vi "Acquiring.vi"(4 "Notify":refnum<notifier>, 6 "GrphChrt Refnum":refnum<vi>, 8 "error in":errorcluster, 9 "Processing Queue":refnum<queue>, 10 "Flow Queue":refnum<queue>, 11 "Acquire Queue":refnum<queue>) -> (0 "error out":errorcluster)   [LabVIEW 2016]
uses:
  Queue Message Handler/Message Cluster.ctl
  Control/Settings.ctl
  Control/port config.ctl
  <vilib>/LabVIEW Interface for Arduino/Type Defs/Board Type.ctl
  <vilib>/LabVIEW Interface for Arduino/Type Defs/Arduino Resource.ctl
  Queue Message Handler/Message Queue.lvlib
  <vilib>/LabVIEW Interface for Arduino/LabVIEW Interface for Arduino.lvlib
panel:
  out "delta t":dbl
  out "Waveform Chart":dbl[](graph)
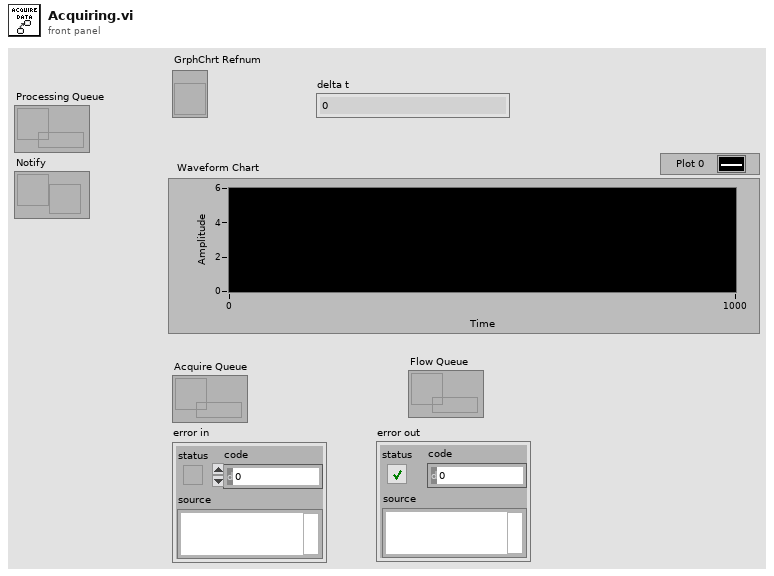
[diagram p1: front panel]
types:
  T1 = typedef "Settings.ctl" = cluster{"Port":T2, "Sample Rate (HZ)":u16, "Samples to Read":u16, "Input Pin":u8, "File path saved":path}
  T2 = typedef "port config.ctl" = cluster{"Port Name":refnum<visa-resource-name>, "Board Type":T3, "Baud Rate":u32}
  T3 = typedef "LabVIEW Interface for Arduino.lvlib/Board Type.ctl" = enum16{"Uno", "Dimuelanove w/Atmega 328", "Mega 2560"}
  T4 = typedef "LabVIEW Interface for Arduino.lvlib/Arduino Resource.ctl" = cluster{"VISA resource":refnum<visa-resource-name>, "Board Type":T3, "Connection Type":enum8{"USB / Serial"}, "Bytes Per Packet (15)":u8}
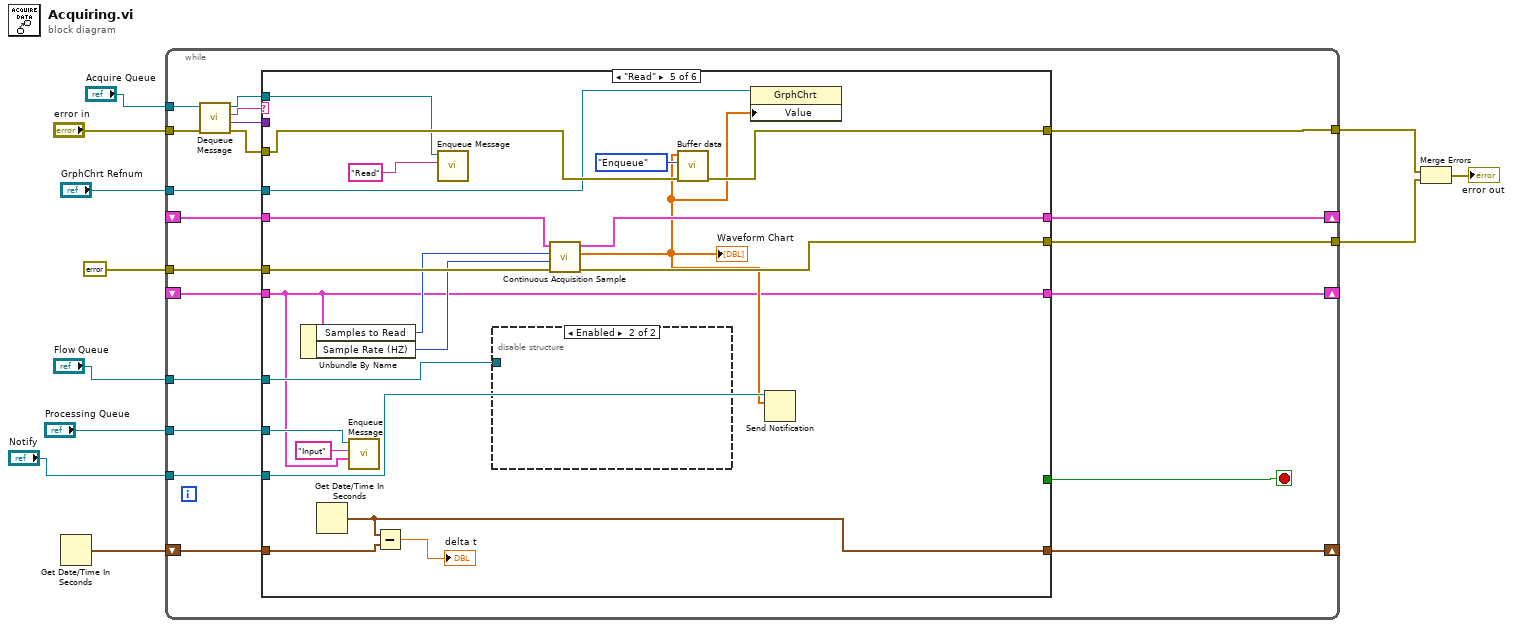
[diagram p0: block diagram]
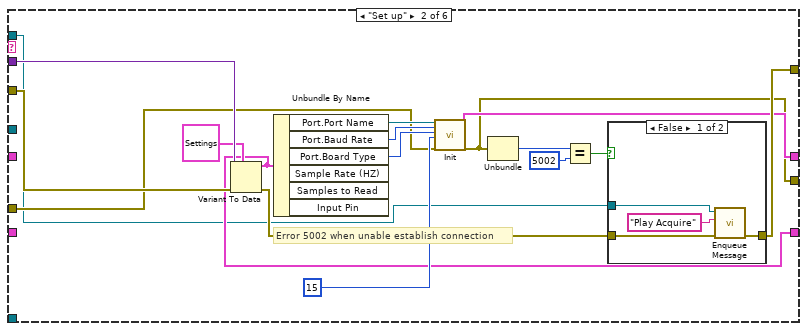
[diagram p3: hidden frame]
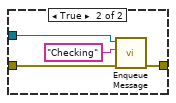
[diagram p4: hidden frame]
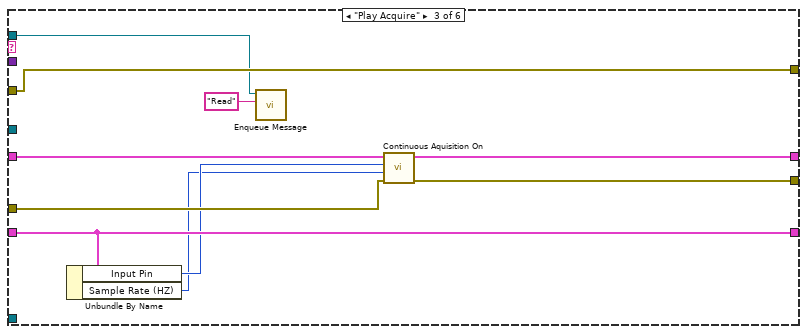
[diagram p5: hidden frame]
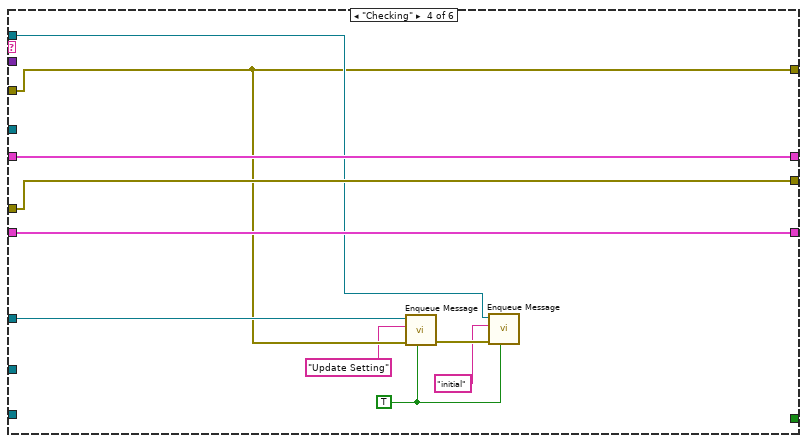
[diagram p6: hidden frame]
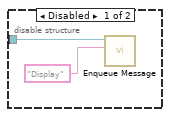
[diagram p7: hidden frame]
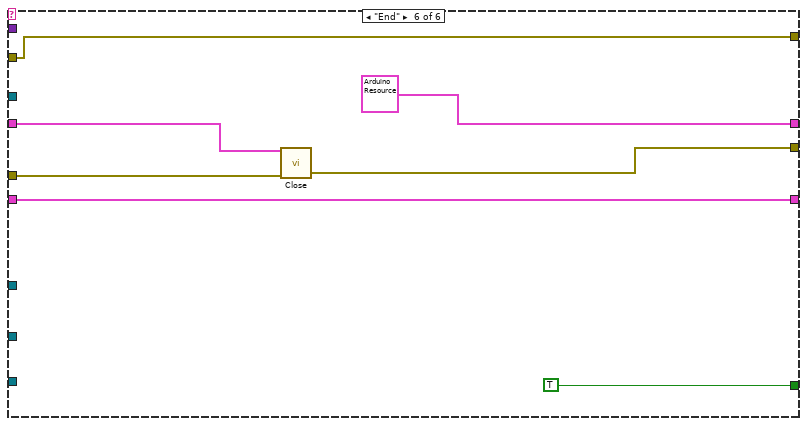
[diagram p8: hidden frame]
diagram:
  n1 = Get Date/Time In Seconds() -> (seconds since 1Jan1904=w1:timestamp)
  n2 = while {
    tunnel: "Acquire Queue" -> [w31]
    tunnel: "error in" -> [w30]
    shift-right: [w25] -> _
    shift-left: _ -> [w24]
    tunnel: [w23] -> w7
    tunnel: errorcluster {"status"=FALSE, "code"=0, "source"=""} ("error in") -> [w22]
    tunnel: [w20] -> w8
    shift-right: [w19] -> _
    shift-left: _ -> [w18]
    tunnel: "Flow Queue" -> [w17]
    tunnel: "GrphChrt Refnum" -> [w16]
    tunnel: "Processing Queue" -> [w15]
    tunnel: "Notify" -> [w14]
    shift-right: [w12] -> _
    shift-left: w1 -> [w13]
    stop <- w28 stop-if-true
    n3 = call "Dequeue Message.vi"("error in (no error)"=w30, "Message Queue"=w31) -> ("error out"=w26:errorcluster, "Message Data"=w27:variant, "Message"=w29:string, "dup Message Queue"=w21:refnum<queue>)  [unwired: 6 in]
    n4 = case shown="\"Read\"" w29 {
      tunnel: [_ _ _ _ _ TRUE] -> w28
      tunnel: w27 -> [_ w52 _ _ _ _]
      tunnel: w26 -> [w33 w46 w70 w75 w94 w109]
      tunnel: [w35 w37 w66 w78 w98 T4 {"VISA resource"="", "Board Type"=enum."Uno", "Connection Type"=enum."USB / Serial", "Bytes Per Packet (15)"=15} ("Arduino Resource")] -> w25
      tunnel: w24 -> [w35 _ w67 w78 w99 w105]
      tunnel: [w34 w36 w64 w80 w100 w106] -> w23
      tunnel: w22 -> [w34 w45 w65 w80 w101 w107]
      tunnel: w21 -> [_ w39 w69 w77 w91 _]
      tunnel: [w33 w38 w70 w75 w93 w109] -> w20
      tunnel: [w32 w44 w63 w79 w81 w108] -> w19
      tunnel: w18 -> [w32 _ w63 w79 w81 w108]
      tunnel: w17 -> [_ _ _ w76 w90 _]
      tunnel: w16 -> [_ _ _ _ w89 _]
      tunnel: w15 -> [_ _ _ _ w88 _]
      tunnel: w14 -> [_ _ _ _ w86 _]
      tunnel: w13 -> [_ _ _ _ w84 _]
      tunnel: [_ _ _ _ w83 _] -> w12
      frame "initial", Default {
      }
      frame "Set up" {
        # "Error 5002 when unable establish connection"
        n5 = Variant To Data(error in=w46, type=T1 {"Port"={"Port Name"="", "Board Type"=enum."Uno", "Baud Rate"=115200}, "Sample Rate (HZ)"=100, "Samples to Read"=50, "Input Pin"=0, "File path saved"=path ""} ("Settings out"), Variant=w52) -> (data=w44:T1, error out=w40:errorcluster)
        n6 = Unbundle By Name(w44) -> ("Port.Port Name"=w50:refnum<visa-resource-name>, "Port.Baud Rate"=w49:u32, "Port.Board Type"=w48:T3)  [unwired: 3 out]
        n7 = call <vilib>:"Init.vi"("VISA resource"=w50, "Baud Rate (115200)"=w49, "Board Type (Uno)"=w48, "Bytes Per Packet (15)"=u32 15, "error in"=w45) -> ("Arduino Resource"=w37:T4, "error out"=w36:errorcluster)  [unwired: 13 in]
        n8 = Unbundle(w36) -> ("code"=w43:i32)  [unwired: 2 out]
        n9 = Equal?(x=w43, y=5002) -> (x = y?=w41:bool)
        n10 = case shown="False" w41 {
          tunnel: w40 -> [w54 w59]
          tunnel: w39 -> [w56 w58]
          tunnel: [w53 w57] -> w38
          frame False {
            n11 = call "Enqueue Message.vi"("error in (no error)"=w54, "Message"="Play Acquire", "Message Queue"=w56) -> ("error out"=w53:errorcluster)  [unwired: 7 in, 1 out]
          }
          frame True {
            n12 = call "Enqueue Message.vi"("error in (no error)"=w59, "Message"="Checking", "Message Queue"=w58) -> ("error out"=w57:errorcluster)  [unwired: 7 in, 1 out]
          }
        }
      }
      frame "Play Acquire" {
        n13 = Unbundle By Name(w63) -> ("Input Pin"=w62:u8, "Sample Rate (HZ)"=w61:u16)
        n14 = call "Enqueue Message.vi"("Message"="Read", "Message Queue"=w69) -> ()  [unwired: 8 in, 2 out]
        n15 = call <vilib>:"Continuous Aquisition On.vi"("error in"=w65, "Acquition Speed"=w61, "Analog Input Pin"=w62, "Arduino Resource"=w67) -> ("error out"=w64:errorcluster, "Arduino Resource"=w66:T4)  [unwired: 6 in]
      }
      frame "Checking" {
        w71 = TRUE ("Priority Message? (F)")
        n16 = call "Enqueue Message.vi"("Priority Message? (F)"=w71, "error in (no error)"=w75, "Message"="Update Setting", "Message Queue"=w76) -> ("error out"=w73:errorcluster)  [unwired: 6 in, 1 out]
        n17 = call "Enqueue Message.vi"("Priority Message? (F)"=w71, "error in (no error)"=w73, "Message"="initial", "Message Queue"=w77) -> ()  [unwired: 6 in, 2 out]
      }
      frame "Read" {
        n18 = Unbundle By Name(w81) -> ("Samples to Read"=w97:u16, "Sample Rate (HZ)"=w96:u16)
        n19 = Get Date/Time In Seconds() -> (seconds since 1Jan1904=w83:timestamp)
        n20 = call "Enqueue Message.vi"("Message Data"=w81, "Message"="Input", "Message Queue"=w88) -> ()  [unwired: 7 in, 2 out]
        n21 = Subtract(x=w83, y=w84) -> (x-y=→"delta t":dbl)
        n22 = call "Enqueue Message.vi"("Message"="Read", "Message Queue"=w91) -> ()  [unwired: 8 in, 2 out]
        n23 = disable-structure shown="Enabled" {
          disable-tunnel: w90 -> [w103 _]
          frame Disabled {
            n24 = call "Enqueue Message.vi"("Message"="Display", "Message Queue"=w103) -> ()  [unwired: 8 in, 2 out]
          }
          frame Enabled {
          }
        }
        n25 = call <vilib>:"Continuous Acquisition Sample.vi"("Arduino Resource"=w99, "Samples to Read"=w97, "Sample Rate (HZ)"=w96, "error in (no error)"=w101) -> ("Arduino Resource"=w98:T4, "Data"=w85:dbl[], "error out"=w100:errorcluster)  [unwired: 4 in]
        "Waveform Chart" <- w85
        n26 = call "Buffer data.vi"("Error in"=w94, "Command"=enum16{"Create", "Enqueue", "Dequeue", "Clear"}."Enqueue", "Data In"=w85) -> ("error out"=w93:errorcluster)  [unwired: 7 in, 1 out]
        n27 = property class="GrphChrt"(reference=w89, "Value"=w85) -> ()  [unwired: 1 in, 2 out]
        n28 = Send Notification(notification=w85, notifier=w86) -> ()  [unwired: 1 in, 2 out]
      }
      frame "End" {
        n29 = call <vilib>:"Close.vi"("Arduino Resource"=w105, "error in"=w107) -> ("error out"=w106:errorcluster)  [unwired: 13 in]
      }
    }
  }
  n30 = Merge Errors(w8, w7) -> (→"error out":errorcluster)
